vi "Main.vi"() -> ()   [LabVIEW 2015]
uses:
  read_info_ctrl.ctl
panel:
  in  "?":T1(tab)
  in  "VM Name":u16(ring) items=["rtatsvm-1", "rtatsvm-2", "rtatsvm-3", "RTATSVM-4", "rtatsvm-5", "RTATSVm-6", "rtatsvm-7", "rtatsvm-8", "rtatsvm-9", "RTATSVM-10", "rtatsvm-11", "rtatsvm-12", "rtvm-1", "rtvm-2", "rtvm-3", "rtvm-4", "rtvm-5", "rtvm-6", "rtvm-7"]
  out "Selected VM":string
  in  "Trigger":bool
  out "error out":errorcluster
  out "Status OF the Target":bool
  in  "Enable E-Mail":bool
  in  "Listbox Target":i32[](listbox)
  in  "LabView Version":u16(ring) items=["2018SP1", "2019   "]
  in  "LabView Version File":path=path "C:/Weekly Runs/Weekly_runs_General/Select_verison.txt"
  in  "Target File Path":path=path "C:/Weekly Runs/Weekly_runs_General/rt_target.txt"
  in  "Log file path":path=path "C:/Weekly Runs/Weekly_runs_General/Log/log.txt"
  in  "Generated ini location path":string="C:\\Weekly Runs\\Generated ini\\"
  in  "OS Specific path":T2(array[cluster])
  in  "General INI path":path=path "C:/Weekly Runs/Weekly_runs_General/general.ini"
  in  "Avaliable target xml files":path=path "C:/Weekly Runs/Weekly_runs_General/Xml files of target"
  in  "Report XML File path":path=path "C:/Weekly Runs/Weekly_runs_General"
  in  "Basic input cammand":string="perl vmware-cmd.pl -H 10.164.43.31 -U root -P INpwdAdm!n \""
  in  "VM's path":path=path "C:/Weekly Runs/Weekly_runs_General/rt_vm.txt"
  in  "Basic  vSphere Path":path=path "C:/Program Files (x86)/VMware/VMware vSphere CLI/bin"
  in  "Sefix Like Softe rest /\" revertsnapshot":string="\" revertsnapshot"
  out "standard output":string
  out "standard error":string
  out "concatenated Cammand":string
  in  "Sefix Restart":string="\" reset soft"
  in  "Mail Server":string="mailout.natinst.com"
  in  "Subject  For Email":string="Weekly Runs"
  out "invalid recipients":string[](array[string])
  in  "TO: [Mail_Reciepient]":string[](array[string])
  out "Body Of E-mail":string
  in  "From [Sender Email]":string="Weekly@ni.com"
  # "Weekly Runs VI 2.0"
  # "This VI is created to Trigger Weekly Runs\n\nThe VI Working Directory is \"C:\\Weekly Runs\\AWRT\" \nThere are few folder and Files that need to create\n   C:\\Weekly Runs\\AWRT\\Weekly_runs_General \n       Note: That this is the location for all OS General.ini files has to be located\n    and a file rt_target.txt which contain RT target Details like\n         Syntax:  RT_Target_Name:OS_Type:filter_.txt:avoid.txt\n           Example: RT-cRIO-9014--2:VxWorks:filter_rtats-crio-9014.txt:avoid_rtats-crio-9014.txt\n    and also a file rt_vm.txt which contain the VM details\n          Syntax:  VM's Name:VMXpath:OS: Bitness\n            Example :rtatsvm-1:/vmfs/volumes/4f4fc760-e56c6c04-9603-d067e5fc28e5/rtatsvm-1/rtatsvm-1.vmx:win 7 SP1:32 \n\ngeneral.ini contains 1st half of the script its generally installation steps.\npharlap.ini/VxWorks.ini/ARM.ini/x64.ini is the 2nd half the trigger the RTATS Steps\n\nFew common terminology used\n$test_names           contains the test step\n$test_definitions     contains the execution step\nBITTest               32/64\nPROGRAM_FILE_TYPE     Program Files (x86)/Program Files\nTargerNAME          Target actual Name like [RT-pxi-8110-1]\n$AVOID            Like avoid_rtats-crio-9068.txt\n$FILTER            like filter_rtats-crio-9068.txt\nLV_VERSION             labview Versions like 2018,2018 SP1,2019\n\n\n\nThis is finally Edited by Hemanth Kothari[hemanth.kumar.kothari@ni.com]"
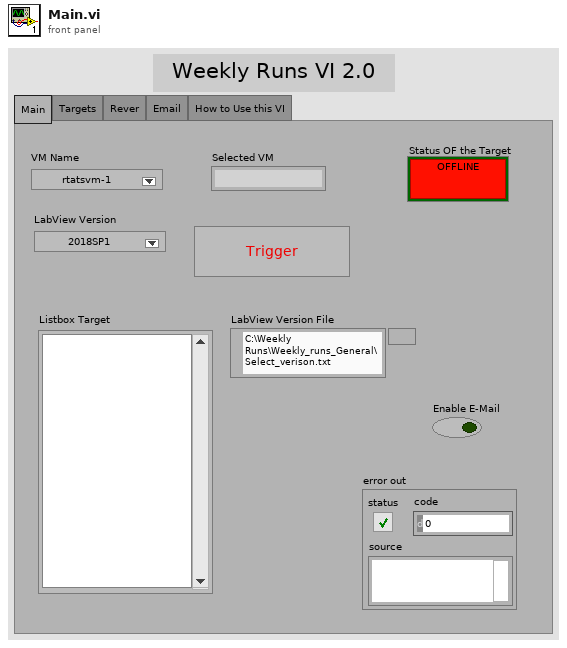
[diagram p1: front panel]
types:
  T1 = enum32{"Main", "Targets", "Rever", "Email", "How to Use this VI"}
  T2 = cluster{"OS Name":string, "OS Specific General  ini":path}[]
  T3 = typedef "read_info_ctrl.ctl" = enum16{"Initialize VM", "Initialize Target", "wait for user input", "Revert VM", "Restart", "Stop"}
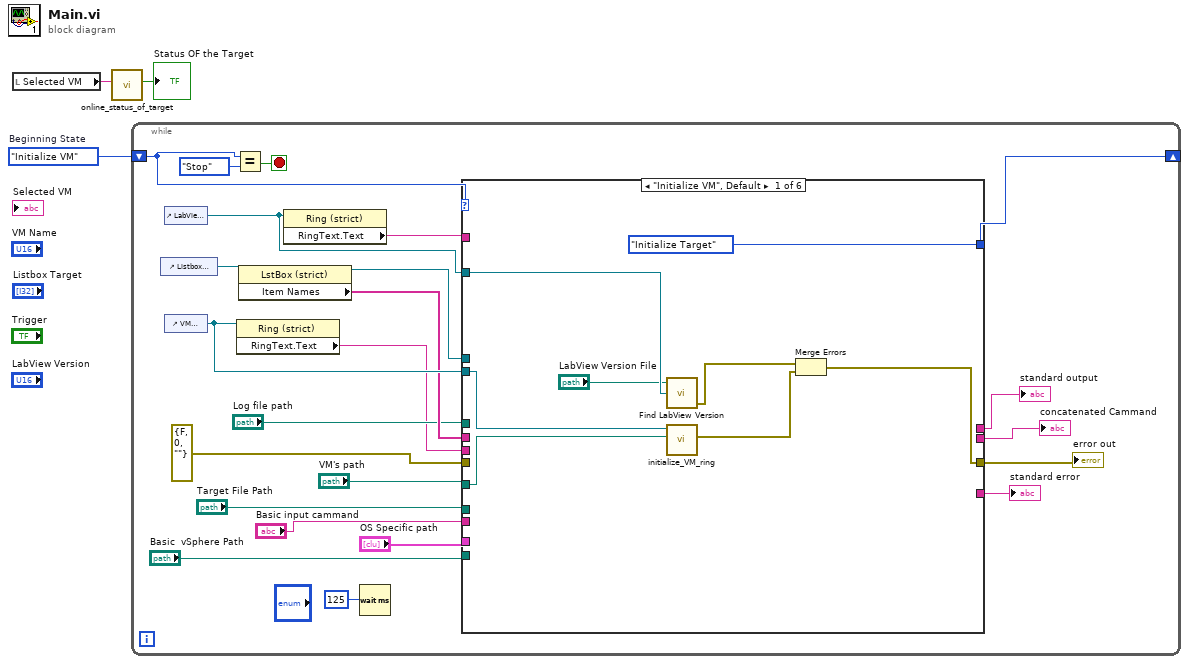
[diagram p0: block diagram]
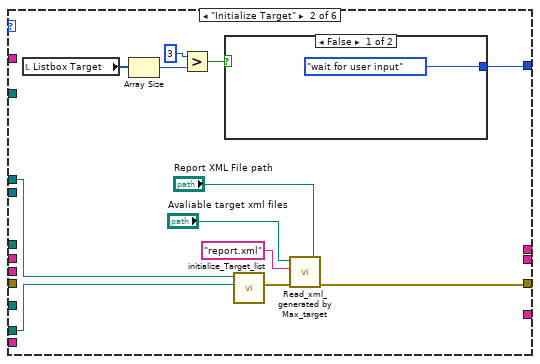
[diagram p2: hidden frame]
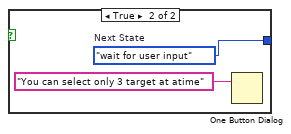
[diagram p3: hidden frame]
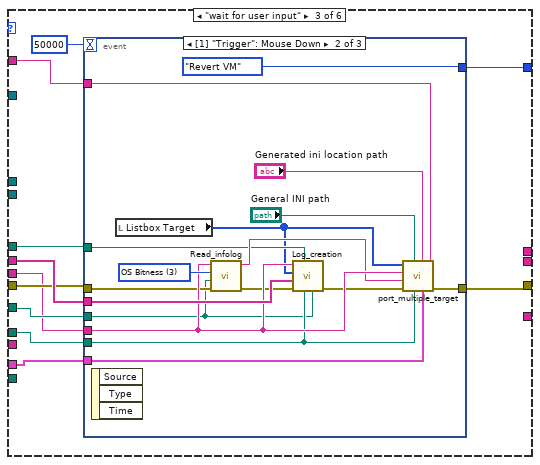
[diagram p4: hidden frame]
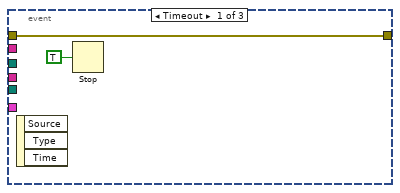
[diagram p5: hidden frame]
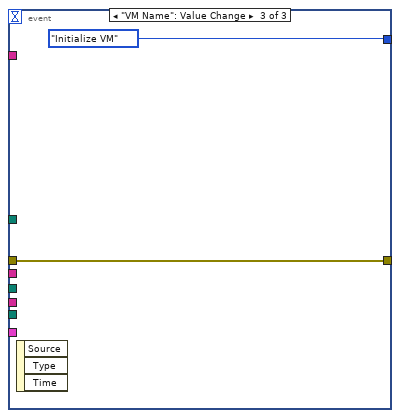
[diagram p6: hidden frame]
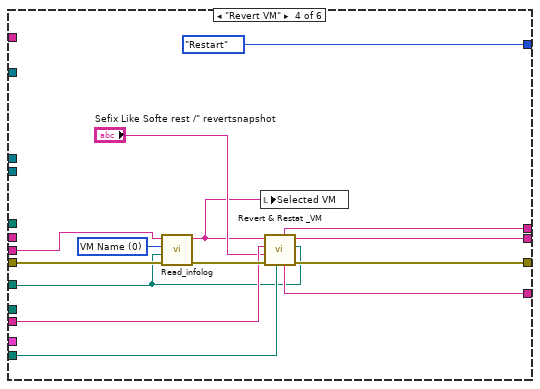
[diagram p7: hidden frame]
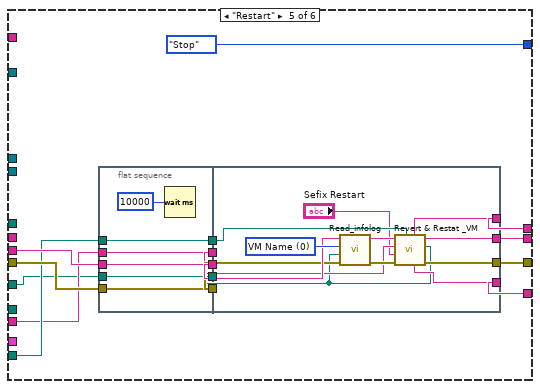
[diagram p8: hidden frame]
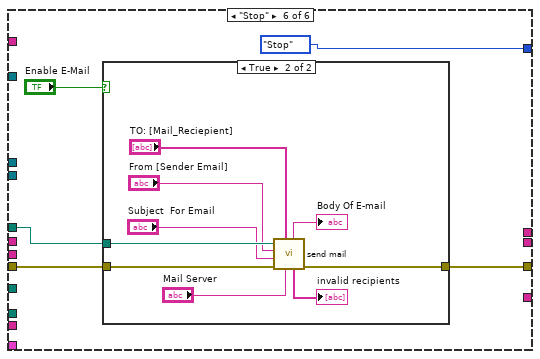
[diagram p9: hidden frame]
diagram:
  w1 = read_info_ctrl."Initialize VM"  # Beginning State
  n1 = local read "Selected VM"() -> (w3:string)
  n2 = call "online_status_of_target.vi"("String"=w3) -> ("x >= 0?"=→"Status OF the Target":bool)  [unwired: 9 in, 1 out]
  n3 = while {
    shift-right: [w9] -> _
    shift-left: w1 -> [w8]
    stop <- w26 stop-if-true
    n4 = control-ref of="Listbox Target"() -> (w7:refnum<vi>)
    n5 = control-ref of="LabView Version"() -> (w4:refnum<vi>)
    n6 = control-ref of="VM Name"() -> (w19:refnum<vi>)
    n7 = Equal?(x=w8, y=read_info_ctrl."Stop" ("States")) -> (x = y?=w26:bool)
    n8 = property class="Ring (strict)"(reference=w19) -> ("RingText.Text"=w6:string)  [unwired: 1 in, 2 out]
    n9 = property class="LstBox (strict)"(reference=w7) -> (reference out=w16:refnum<vi>, "Item Names"=w18:string[])  [unwired: 1 in, 1 out]
    n10 = property class="Ring (strict)"(reference=w4) -> ("RingText.Text"=w5:string)  [unwired: 1 in, 2 out]
    n11 = Wait (ms)(milliseconds to wait=u32 125) -> ()  [unwired: 1 out]
    n12 = case shown="\"Initialize VM\", Default" w8 {
      tunnel: [read_info_ctrl."Initialize Target" ("Next State") w40 w60 read_info_ctrl."Restart" ("Next State") read_info_ctrl."Stop" ("Next State") read_info_ctrl."Stop" ("Next State")] -> w9
      tunnel: errorcluster {"status"=FALSE, "code"=0, "source"=""} ("error in (no error)") -> [_ _ w57 w93 w108 w133]
      tunnel: [w27 w36 w53 w84 w107 w130] -> w24
      tunnel: w19 -> [w33 _ _ _ _ _]
      tunnel: w6 -> [_ _ w52 w94 w109 _]
      tunnel: w16 -> [_ w42 _ _ _ _]
      tunnel: w18 -> [_ _ w58 _ _ _]
      tunnel: "Target File Path" -> [_ w41 w51 _ _ _]
      tunnel: "VM's path" -> [w32 _ w55 w83 w102 _]
      tunnel: "Log file path" -> [_ _ w56 _ _ w131]
      tunnel: "Basic  vSphere Path" -> [_ _ _ w86 w106 _]
      tunnel: "Basic input cammand" -> [_ _ _ w91 w105 _]
      tunnel: [_ _ _ w90 w104 _] -> w11
      tunnel: [_ _ _ w89 w103 _] -> w22
      tunnel: [_ _ _ w88 w96 _] -> w21
      tunnel: "OS Specific path" -> [_ _ w54 _ _ _]
      tunnel: w5 -> [_ _ w50 _ _ _]
      tunnel: w4 -> [w31 _ _ _ _ _]
      frame "Initialize VM", Default {
        n13 = call "Find LabView Version.vi"("Lv version"=w31, "LabView Version File"="LabView Version File") -> ("error out"=w29:errorcluster)  [unwired: 3 in]
        n14 = call "initialize_VM_ring.vi"("VM's path"=w32, "Ring in"=w33) -> ("error out"=w28:errorcluster)  [unwired: 9 in]
        n15 = Merge Errors(w29, w28) -> (w27:errorcluster)
      }
      frame "Initialize Target" {
        n16 = local read "Listbox Target"() -> (w46:i32[])
        n17 = Array Size(array=w46) -> (size(s)=w44:i32)
        n18 = Greater?(x=3, y=w44) -> (0:w43:bool)
        n19 = case shown="False" w43 {
          tunnel: [read_info_ctrl."wait for user input" ("Next State") w48] -> w40
          frame False {
          }
          frame True {
            w48 = read_info_ctrl."wait for user input"  # Next State
            n20 = One Button Dialog(message="You can select only 3 target at atime") -> ()  [unwired: 1 in, 1 out]
          }
        }
        n21 = call "initialize_Target_list.vi"("Target File Path"=w41, "reference"=w42) -> ("error out"=w35:errorcluster)  [unwired: 9 in]
        n22 = call "Read_xml_generated by Max_target.vi"("Report XML File path"="Report XML File path", "error in (no error)"=w35, "Name of the file"="report.xml", "Avaliable target xml files"="Avaliable target xml files") -> ("error out"=w36:errorcluster)  [unwired: 1 in, 2 out]
      }
      frame "wait for user input" {
        n23 = event shown="[1] \"Trigger\": Mouse Down" {
          selector: _ -> [_ _ _]
          dyn-events: _ -> [_ _ _]
          timeout: 50000 -> [_ _ _]
          tunnel: [_ read_info_ctrl."Revert VM" ("Next State") read_info_ctrl."Initialize VM" ("Next State")] -> w60
          tunnel: w52 -> [_ w77 _]
          tunnel: w58 -> [_ w78 _]
          tunnel: [w61 w68 w80] -> w53
          tunnel: w57 -> [w61 w75 w80]
          tunnel: w56 -> [_ w74 _]
          tunnel: w55 -> [_ w70 _]
          tunnel: w51 -> [_ w71 _]
          tunnel: w54 -> [_ w69 _]
          tunnel: w50 -> [_ w63 _]
          event Timeout {
            n24 = event-data() -> ()  [unwired: 1 in, 3 out]
            n25 = Stop(stop? (T)=TRUE) -> ()
          }
          event "Trigger": Mouse Down {
            w79 = u16 3 items=["VM Name", "VMX Path", "OS Detail", "OS Bitness"] ("Ring")
            n26 = event-data() -> ()  [unwired: 1 in, 3 out]
            n27 = local read "Listbox Target"() -> (w64:i32[])
            n28 = call "Read_infolog.vi"("vm name"=w77, "Details of vm"=w79, "VM's path"=w70, "error in"=w75) -> ("VMX Path details"=w76:string, "error out"=w66:errorcluster)  [unwired: 5 in]
            n29 = call "Log_creation.vi"("VM's path"=w70, "Target File Path"=w71, "Log file path"=w74, "error in"=w66, "Item Names"=w78, "Listbox Target"=w64, "VM name"=w77) -> ("error out"=w67:errorcluster)  [unwired: 4 in]
            n30 = call "port_multiple_target.vi"("LV Version"=w63, "OS Specific path"=w69, "Generated ini location path"="Generated ini location path", "Target File Path"=w71, "General INI path"="General INI path", "error in"=w67, "Bitness"=w76, "VM Name"=w77, "Listbox  Target"=w64) -> ("error out"=w68:errorcluster)  [unwired: 2 in]
          }
          event "VM Name": Value Change {
            n31 = event-data() -> ()  [unwired: 1 in, 3 out]
          }
        }
      }
      frame "Revert VM" {
        w95 = u16 0 items=["VM Name", "VMX Path", "OS Detail", "OS Bitness"] ("Ring")
        n32 = call "Read_infolog.vi"("vm name"=w94, "Details of vm"=w95, "VM's path"=w83, "error in"=w93) -> ("VMX Path details"=w82:string, "error out"=w92:errorcluster)  [unwired: 5 in]
        n33 = local write "Selected VM"(w82) -> ()
        n34 = call "Revert & Restat _VM.vi"("VM Name"=w82, "Basic input cammand"=w91, "Sefix Like Softe rest/\" revertsnapshot"="Sefix Like Softe rest /\" revertsnapshot", "error in (no error)"=w92, "Basic  vSphere Path"=w86, "VM's path"=w83) -> ("standard output"=w90:string, "standard error"=w89:string, "concatenated Cammand"=w88:string, "error out"=w84:errorcluster)  [unwired: 1 in]
      }
      frame "Restart" {
        n35 = flat-sequence {
          tunnel: w102 -> [w112]
          tunnel: w105 -> [w113]
          tunnel: w106 -> [w114]
          tunnel: w108 -> [w115]
          tunnel: w109 -> [w116]
          tunnel: [w116] -> w101
          tunnel: [w115] -> w100
          tunnel: [w114] -> w99
          tunnel: [w113] -> w98
          tunnel: [w112] -> w97
          tunnel: [w124] -> w107
          tunnel: [w120] -> w104
          tunnel: [w119] -> w103
          tunnel: [w118] -> w96
          tunnel: w101 -> [w128]
          tunnel: w100 -> [w127]
          tunnel: w99 -> [w123]
          tunnel: w98 -> [w122]
          tunnel: w97 -> [w117]
          frame #0 {
            n36 = Wait (ms)(milliseconds to wait=u32 10000) -> ()  [unwired: 1 out]
          }
          frame #1 {
            w129 = u16 0 items=["VM Name", "VMX Path", "OS Detail", "OS Bitness"] ("Ring")
            n37 = call "Read_infolog.vi"("vm name"=w128, "Details of vm"=w129, "VM's path"=w117, "error in"=w127) -> ("VMX Path details"=w126:string, "error out"=w125:errorcluster)  [unwired: 5 in]
            n38 = call "Revert & Restat _VM.vi"("VM Name"=w126, "Basic input cammand"=w122, "Sefix Like Softe rest/\" revertsnapshot"="Sefix Restart", "error in (no error)"=w125, "Basic  vSphere Path"=w123, "VM's path"=w117) -> ("standard output"=w120:string, "standard error"=w119:string, "concatenated Cammand"=w118:string, "error out"=w124:errorcluster)  [unwired: 1 in]
          }
        }
      }
      frame "Stop" {
        n39 = case shown="True" "Enable E-Mail" {
          tunnel: [w135 w144] -> w130
          tunnel: w131 -> [_ w143]
          tunnel: w133 -> [w135 w138]
          frame False {
          }
          frame True {
            n40 = call "send mail.vi"("Mail Server"="Mail Server", "TO: [Mail_Reciepient]"="TO: [Mail_Reciepient]", "error in"=w138, "Subject  For Email"="Subject  For Email", "From [Sender Email]"="From [Sender Email]", "LogFile path"=w143) -> ("error out"=w144:errorcluster, "invalid recipients"=→"invalid recipients":string[], "Body Of E-mail"=→"Body Of E-mail":string)  [unwired: 3 in]
          }
        }
      }
    }
    "error out" <- w24
    "standard output" <- w11
    "standard error" <- w22
    "concatenated Cammand" <- w21
  }
